vi "Build Array of Type in Variant.vi"(5 "error in":errorcluster, 7 "Type in":variant) -> (1 "error out":errorcluster, 3 "Array of \"Type in\"":variant)   [LabVIEW 2025, in "XNode Support.lvlib"]
uses:
  XNode Support.lvlib
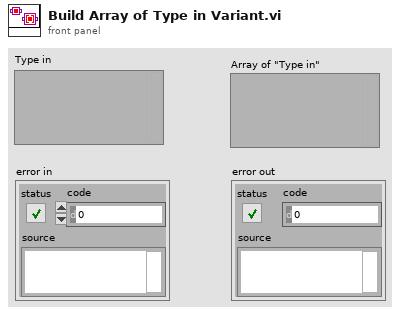
[diagram p1: front panel]
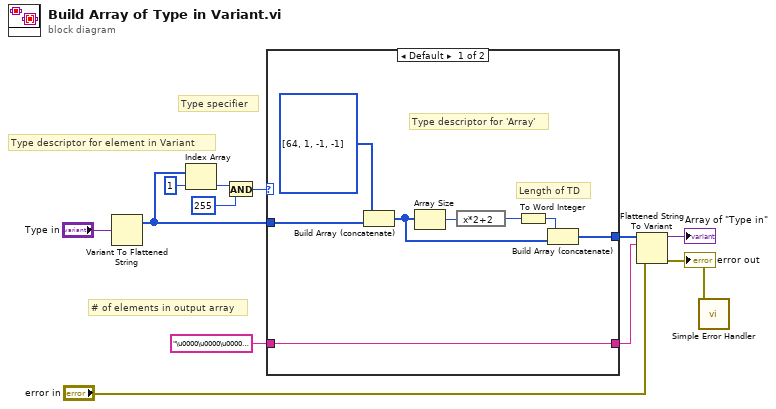
[diagram p0: block diagram]
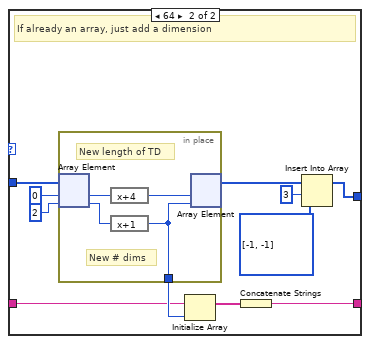
[diagram p2: hidden frame]
diagram:
  # "Type specifier"
  # "# of elements in output array"
  # "Type descriptor for element in Variant"
  n1 = Variant To Flattened String(Variant="Type in") -> (1:w8:i16[])  [unwired: 1 out]
  n2 = Index Array(array=w8, index=1) -> (element=w11:i16)
  n3 = And(x=w11, y=i16 255) -> (x .and. y?=w10:i16)
  n4 = case shown="Default" w10 {
    tunnel: [w16 w31] -> w7
    tunnel: w8 -> [w14 w22]
    tunnel: [w13 w26] -> w6
    tunnel: "\u0000\u0000\u0000\u0000" ("data string 2") -> [w13 w25]
    frame Default {
      # "Length of TD"
      # "Type descriptor for 'Array'"
      n5 = Build Array (concatenate)(i16[] [64, 1, -1, -1] ("type string 2"), w14) -> (w17:i16[])
      n6 = Array Size(array=w17) -> (size(s)=w19:i32)
      n7 = expression code="x*2+2"(w19) -> (w18:i32)
      n8 = To Word Integer(number=w18) -> (16bit integer=w15:i16)
      n9 = Build Array (concatenate)(w15, w17) -> (w16:i16[])
    }
    frame 64 {
      # "If already an array, just add a dimension"
      n10 = in-place {
        in-place-border: [w32] -> w28
        # "New # dims"
        # "New length of TD"
        n11 = in-place-array #1(w22, 0, 2) -> (w35:i16, w34:i16)
        n12 = expression code="x+4"(w35) -> (w33:i16)
        n13 = expression code="x+1"(w34) -> (w32:i16)
        n14 = in-place-array #1(w33, w32) -> (w21:i16[])  [unwired: 2 out]
      }
      n15 = Initialize Array(w25, w28) -> (w27:string[])
      n16 = Concatenate Strings(w27) -> (w26:string)
      n17 = Insert Into Array(array=w21, index=3, new element=i16[] [-1, -1] ("output array")) -> (w31:i16[])
    }
  }
  n18 = Flattened String To Variant(4:"error in", 6:w6, 7:w7) -> (0:w1:errorcluster, 3:→"Array of \"Type in\"":variant)
  "error out" <- w1
  n19 = call <vilib>:"Simple Error Handler.vi"("error in (no error)"=w1) -> ()  [unwired: 4 in, 5 out]
